vi "Run Client.vi"() -> ()   [LabVIEW 2020, in "Client.lvlib"]
uses:
  Client/Client.lvlib
  Measurement Service Client V2/RPC Messages/ni_measurementlink_measurement_v2_MeasureRequest.ctl
  Measurement Service Client V2/RPC Messages/google_protobuf_Any.ctl
  Measurement Service Client V2/RPC Messages/ni_measurementlink_PinMapContext.ctl
  Service/Service/Measurement Results.ctl
  Service/Service/Measurement Configuration.ctl
  045899de-a912-426a-8a5d-a949b9672173.vi
  <vilib>/gRPC/LabVIEW gRPC Library/Server API/Translate Protobuf Error.vi
  <vilib>/AdvancedString/1D String Array to Delimited String.vi
  <vilib>/gRPC/LabVIEW gRPC Library/Server API/Server/Get Server DLL Path.vi
  <vilib>/gRPC/LabVIEW gRPC Library/grpc-lvsupport-release.lvlib
  Measurement Service Client V2/Measurement Service Client V2.lvlib
  Service/Service/Service.lvlib
panel:
  in  "time in seconds":dbl=5.0
  out "random numbers":dbl[](graph)
  out "elapsed time":dbl
  out "status":string
  in  "stop":bool
  out "error out":errorcluster
  in  "service to run":string="ServiceforLabVIEWClient_LabVIEW"
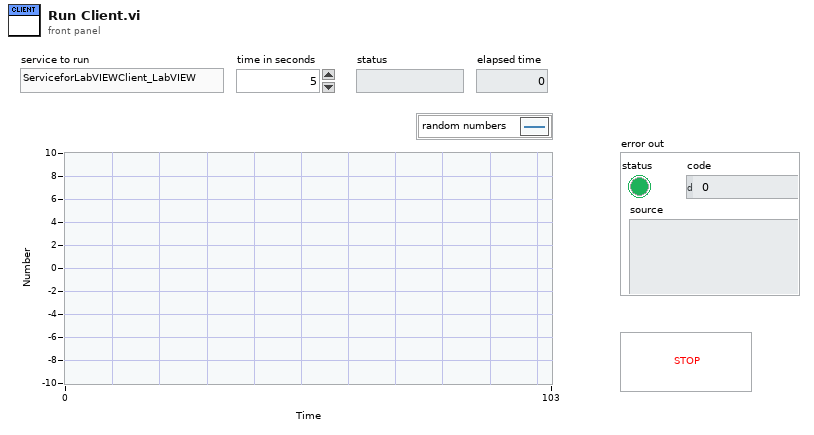
[diagram p1: front panel]
types:
  T1 = typedef "Service.lvlib/Measurement Configuration.ctl" = cluster{"time in seconds":dbl}
  T2 = typedef "Service.lvlib/Measurement Results.ctl" = cluster{"random numbers":dbl[], "status":string, "elapsed time":dbl}
  T3 = typedef "Measurement Service Client V2.lvlib/ni_measurementlink_measurement_v2_MeasureRequest.ctl" = cluster{"configuration_parameters":T4, "pin_map_context":T5}
  T4 = typedef "Measurement Service Client V2.lvlib/google_protobuf_Any.ctl" = cluster{"type_url":string, "value":u8[]}
  T5 = typedef "Measurement Service Client V2.lvlib/ni_measurementlink_PinMapContext.ctl" = cluster{"pin_map_id":string, "sites":i32[]}
  T6 = typedef "grpc-lvsupport-release.lvlib/grpcId.ctl" = u64
  T7 = typedef "grpc-lvsupport-release.lvlib/Message Metadata.ctl" = cluster{"Version":i32, "Name":string, "Type Url":string, "Elements":T8[], "Has Oneof":bool}
  T8 = typedef "grpc-lvsupport-release.lvlib/Message Element Metadata.ctl" = cluster{"Field Name":string, "Embedded Message Name":string, "Protobuf Index":i32, "MessageElementType":T9, "Repeated":bool, "Is in Oneof":bool, "Oneof Container Name":string}
  T9 = typedef "grpc-lvsupport-release.lvlib/Message Element Type.ctl" = enum32{"Int32Value", "FloatValue", "DoubleValue", "BoolValue", "StringValue", "MessageValue", "Int64Value", "UInt32Value", "UInt64Value", "EnumValue", "Bytes", "Fixed64", "Fixed32", "SFixed64", "SFixed32", "SInt64", "SInt32"}
  T10 = typedef "grpc-lvsupport-release.lvlib/Any.ctl" = cluster{"Type Url":string, "Bytes":u8[]}
  T11 = typedef "Measurement Service Client V2.lvlib/ni_measurementlink_measurement_v2_MeasureResponse.ctl" = cluster{"outputs":T4}
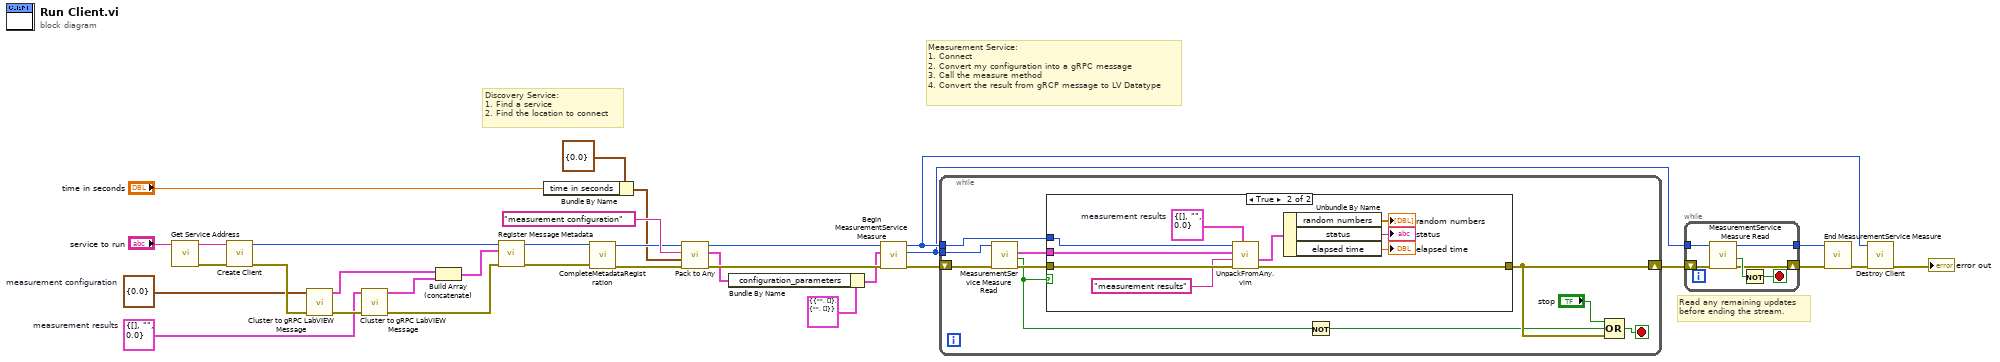
[diagram p0: block diagram]
diagram:
  w4 = T1 {"time in seconds"=0.0}  # measurement configuration
  w9 = T2 {"random numbers"=[], "status"="", "elapsed time"=0.0}  # measurement results
  # "Read any remaining updates \nbefore ending the stream."
  # "Measurement Service:\n1. Connect\n2. Convert my configuration into a gRPC message\n3. Call the measure method\n4. Convert the result from gRCP message to LV Datatype"
  # "Discovery Service:\n1. Find a service\n2. Find the location to connect"
  n1 = call "Get Service Address.vi"("service to run"="service to run") -> ("error out"=w30:errorcluster, "service address"=w14:string)  [unwired: 9 in]
  n2 = call "Create Client.vi"("error in"=w30, "address"=w14) -> ("error out"=w12:errorcluster, "gRPC ID Out"=w29:T6)  [unwired: 8 in]
  n3 = call <vilib>:"Cluster to gRPC LabVIEW Message.vi"("error in"=w12, "Cluster"=w4) -> ("error out"=w11:errorcluster, "gRPC Message Metadata []"=w33:T7[])  [unwired: 7 in, 1 out]
  n4 = call <vilib>:"Cluster to gRPC LabVIEW Message.vi"("error in"=w11, "Cluster"=w9) -> ("error out"=w10:errorcluster, "gRPC Message Metadata []"=w32:T7[])  [unwired: 7 in, 1 out]
  n5 = Build Array (concatenate)(w33, w32) -> (w31:T7[])
  n6 = call <vilib>:"Register Message Metadata.vi"("error in"=w10, "Messages"=w31, "gRPCid in"=w29) -> ("error out"=w26:errorcluster, "gRPCid out"=w27:T6)  [unwired: 7 in]
  n7 = Bundle By Name(cluster=T1 {"time in seconds"=0.0} ("Measurement Configuration"), "time in seconds"="time in seconds") -> (w1:T1)
  n8 = call <vilib>:"CompleteMetadataRegistration.vi"("error in"=w26, "gRPC ID in"=w27) -> ("error out"=w13:errorcluster, "gRPC ID Out"=w24:T6)  [unwired: 8 in]
  n9 = call "Pack to Any.vi"("error in"=w13, "data to pack"=w1, "message type"="measurement configuration" ("Message Type"), "gRPC ID in"=w24) -> ("error out"=w23:errorcluster, "any"=w20:T10, "gRPC ID out"=w22:T6)  [unwired: 5 in]
  n10 = Bundle By Name(cluster=T3 {"configuration_parameters"={"type_url"="", "value"=[]}, "pin_map_context"={"pin_map_id"="", "sites"=[]}} ("Request Data"), "configuration_parameters"=w20) -> (w16:T3)
  n11 = call "Begin MeasurementService Measure.vi"("error in"=w23, "Request Data"=w16, "gRPC ID"=w22) -> ("error out"=w19:errorcluster, "Call Id Out"=w7:T6, "gRPC ID out"=w17:T6)  [unwired: 6 in]
  n12 = while {
    tunnel: w7 -> [w40]
    tunnel: w17 -> [w39]
    shift-right: [w37] -> w8
    shift-left: w19 -> [w41]
    stop <- w43 stop-if-true
    n13 = call "MeasurementService Measure Read.vi"("error in"=w41, "Call ID in"=w40) -> ("error out"=w38:errorcluster, "Success"=w36:bool, "Response Data"=w42:T11)  [unwired: 6 in, 1 out]
    n14 = case shown="True" w36 {
      tunnel: w42 -> [_ w53]
      tunnel: w39 -> [_ w52]
      tunnel: w38 -> [w44 w51]
      tunnel: [w44 w50] -> w37
      frame False {
      }
      frame True {
        w48 = T2 {"random numbers"=[], "status"="", "elapsed time"=0.0}  # measurement results
        n15 = call "UnpackFromAny.vim"("Data Type"=w48, "error in"=w51, "Message Type"="measurement results", "Any"=w53, "gRPCid in"=w52) -> ("error out"=w50:errorcluster, "Unpacked Value"=w54:T2)  [unwired: 4 in, 1 out]
        n16 = Unbundle By Name(w54) -> ("random numbers"=→"random numbers":dbl[], "status"=→"status":string, "elapsed time"=→"elapsed time":dbl)
      }
    }
    n17 = Not(x=w36) -> (.not. x?=w35:bool)
    n18 = Compound Arithmetic op=OR("stop", w35, w37) -> (w43:bool)
  }
  n19 = while {
    tunnel: w7 -> [w57]
    tunnel: [w56] -> w6
    shift-right: [w55] -> w5
    shift-left: w8 -> [w60]
    stop <- w58 stop-if-true
    n20 = call "MeasurementService Measure Read.vi"("error in"=w60, "Call ID in"=w57) -> ("error out"=w55:errorcluster, "Success"=w59:bool, "Call ID"=w56:T6)  [unwired: 6 in, 1 out]
    n21 = Not(x=w59) -> (.not. x?=w58:bool)
  }
  n22 = call "End MeasurementService Measure.vi"("error in"=w5, "Call ID in"=w6) -> ("error out"=w18:errorcluster)  [unwired: 8 in, 1 out]
  n23 = call "Destroy Client.vi"("error in"=w18, "gRPC ID"=w17) -> ("error out"=→"error out":errorcluster)  [unwired: 9 in]
